vi "Q_Driver.vi"(0 "State":string, 2 "Q Name":string, 5 "States[]":string[](array[string]), 11 "Error In":errorcluster, 13 "Operations":T1) -> (4 "Dequeued Ele":string, 15 "Error Out":errorcluster)   [LabVIEW 2020]
uses:
  Typedef's/Q_Operations.ctl
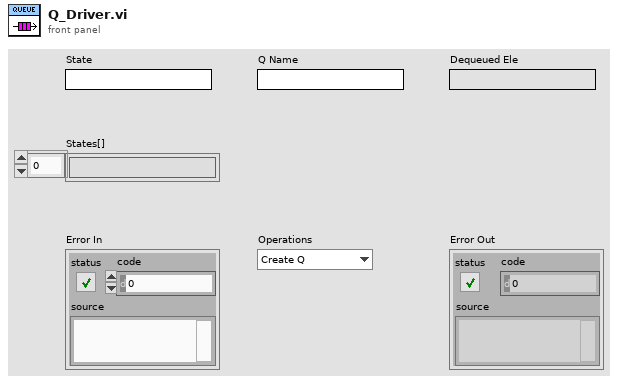
[diagram p1: front panel]
types:
  T1 = typedef "Q_Operations.ctl" = enum16{"Create Q", "Enqueue ", "Dequeue", "Enqueue N ele", "Enstack N ele", "Flush Q", "Destroy Q"}
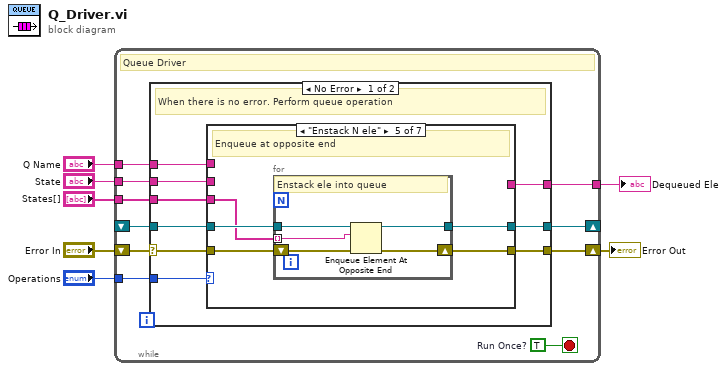
[diagram p0: block diagram]
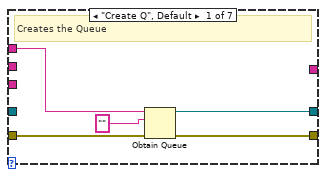
[diagram p2: hidden frame]
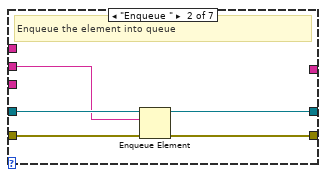
[diagram p3: hidden frame]
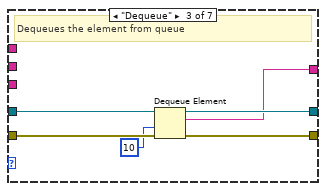
[diagram p4: hidden frame]
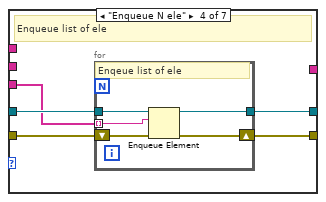
[diagram p5: hidden frame]
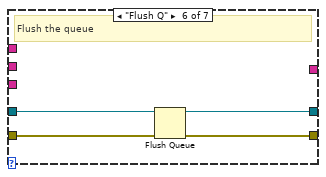
[diagram p6: hidden frame]
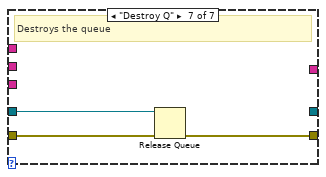
[diagram p7: hidden frame]
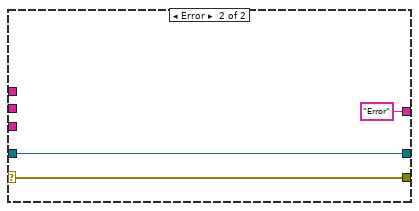
[diagram p8: hidden frame]
diagram:
  n1 = while {
    tunnel: "Operations" -> [w16]
    shift-right: [w14] -> w1
    shift-left: "Error In" -> [w15]
    tunnel: "Q Name" -> [w13]
    shift-right: [w12] -> _
    shift-left: _ -> [w11]
    tunnel: "State" -> [w10]
    tunnel: "States[]" -> [w9]
    tunnel: [w8] -> w2
    stop <- w17 stop-if-true
    w17 = TRUE  # Run Once?
    # "Queue Driver"
    n2 = case shown="No Error" w15 {
      selector: w15 -> [w25 w71]
      tunnel: w16 -> [w26 _]
      tunnel: [w24 w71] -> w14
      tunnel: w13 -> [w23 _]
      tunnel: [w22 w72] -> w12
      tunnel: w11 -> [w21 w72]
      tunnel: w10 -> [w20 _]
      tunnel: w9 -> [w19 _]
      tunnel: [w18 "Error"] -> w8
      frame No Error {
        # "When there is no error. Perform queue operation"
        n3 = case shown="\"Enstack N ele\"" w26 {
          tunnel: w25 -> [w31 w36 w42 w46 w57 w66 w69]
          tunnel: [w30 w35 w41 w47 w56 w65 w68] -> w24
          tunnel: w23 -> [w29 _ _ _ _ _ _]
          tunnel: [w28 w33 w39 w45 w54 w63 _] -> w22
          tunnel: w21 -> [_ w34 w40 w44 w55 w64 w67]
          tunnel: w20 -> [_ w32 _ _ _ _ _]
          tunnel: w19 -> [_ _ _ w43 w53 _ _]
          tunnel: [_ _ w37 _ _ _ _] -> w18
          frame "Create Q", Default {
            # "Creates the Queue"
            n4 = Obtain Queue(name (unnamed)=w29, element data type="", error in (no error)=w31) -> (queue out=w28:refnum<queue>, error out=w30:errorcluster)  [unwired: 2 in, 1 out]
          }
          frame "Enqueue " {
            # "Enqueue the element into queue"
            n5 = Enqueue Element(queue=w34, element=w32, error in (no error)=w36) -> (queue out=w33:refnum<queue>, error out=w35:errorcluster)  [unwired: 1 in, 1 out]
          }
          frame "Dequeue" {
            # "Dequeues the element from queue"
            n6 = Dequeue Element(queue=w40, timeout in ms (-1)=10, error in (no error)=w42) -> (queue out=w39:refnum<queue>, element=w37:string, error out=w41:errorcluster)  [unwired: 1 out]
          }
          frame "Enqueue N ele" {
            # "Enqueue list of ele"
            n7 = for {
              tunnel: [w50] -> w45
              tunnel: w44 -> [w49]
              shift-right: [w52] -> w47
              shift-left: w46 -> [w51]
              tunnel: w43 -> [w48] mode=indexing
              # "Enqeue list of ele"
              n8 = Enqueue Element(queue=w49, element=w48, error in (no error)=w51) -> (queue out=w50:refnum<queue>, error out=w52:errorcluster)  [unwired: 1 in, 1 out]
            }
          }
          frame "Enstack N ele" {
            # "Enqueue at opposite end"
            n9 = for {
              tunnel: w55 -> [w60]
              tunnel: [w59] -> w54
              shift-right: [w61] -> w56
              shift-left: w57 -> [w62]
              tunnel: w53 -> [w58] mode=indexing
              # "Enstack ele into queue"
              n10 = Enqueue Element At Opposite End(queue=w60, element=w58, error in (no error)=w62) -> (queue out=w59:refnum<queue>, error out=w61:errorcluster)  [unwired: 1 in, 1 out]
            }
          }
          frame "Flush Q" {
            # "Flush the queue"
            n11 = Flush Queue(queue=w64, error in (no error)=w66) -> (queue out=w63:refnum<queue>, error out=w65:errorcluster)  [unwired: 1 out]
          }
          frame "Destroy Q" {
            # "Destroys the queue"
            n12 = Release Queue(queue=w67, error in (no error)=w69) -> (error out=w68:errorcluster)  [unwired: 1 in, 2 out]
          }
        }
      }
      frame Error {
      }
    }
  }
  "Dequeued Ele" <- w2
  "Error Out" <- w1
